vi "Remove RTDriver VIs.vi"(8 "error in (no error)":errorcluster, 11 ".NET Refnum in":refnum<k24>) -> (0 "error out":errorcluster, 3 ".NET Refnum out":refnum<k24>)   [LabVIEW 2019, in "TemplatePPL System Explorer.lvlib"]
uses:
  TemplatePPL System Explorer.lvlib
  NationalInstruments.VeriStand.SystemStorage
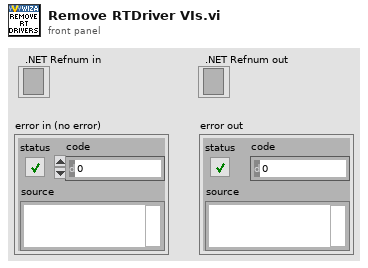
[diagram p1: front panel]
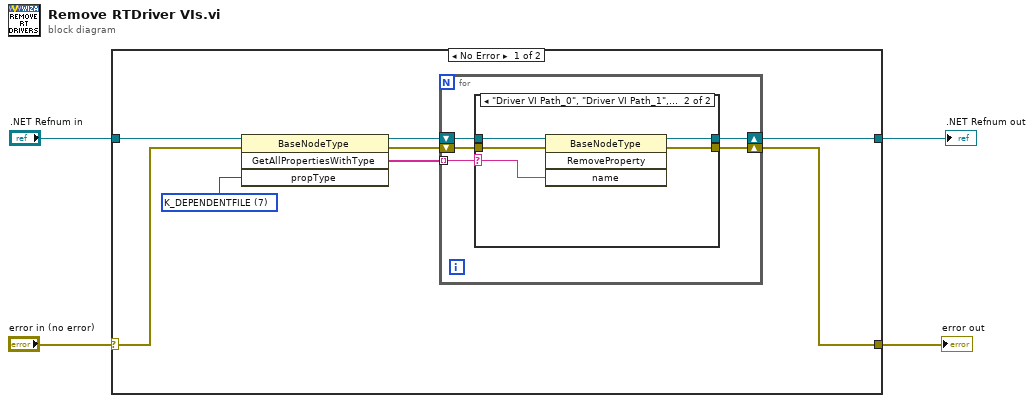
[diagram p0: block diagram]
diagram:
  n1 = case shown="No Error" "error in (no error)" {
    selector: "error in (no error)" -> [w7 w25]
    tunnel: [w12 w25] -> w4
    tunnel: [w11 w26] -> w1
    tunnel: ".NET Refnum in" -> [w8 w26]
    frame No Error {
      w9 = 7 items=["K_STRING", "K_BOOL", "K_I32", "K_U32", "K_DOUBLE", "K_U64", "K_VARIANT", "K_DEPENDENTFILE", "K_DEPENDENTNODE", "K_DATASOURCENODE", "K_U16", "K_DBLARR", "K_U32ARR", "K_I32ARR", "K_STRINGARR", "K_DICTIONARY", "K_DICTIONARYARR", "K_BINARYSTRING", "K_I16", "K_I64", "K_BOOLARR", "K_U64ARR", "K_U16ARR", "K_I64ARR", "K_I16ARR"] ("propType")
      n2 = invoke class="BaseNodeType" method="GetAllPropertiesWithType"(reference=w8, error in=w7, "propType"=w9) -> (reference out=w6:refnum<k24>, error out=w10:errorcluster, "GetAllPropertiesWithType"=w5:string[])  [unwired: 1 in, 1 out]
      n3 = for {
        tunnel: w5 -> [w13] mode=indexing
        shift-right: [w15] -> w12
        shift-left: w10 -> [w16]
        shift-right: [w14] -> w11
        shift-left: w6 -> [w17]
        n4 = case shown="\"Driver VI Path_0\", \"Driver VI Path_1\", \"Driver VI Path_2\", \"Driver VI Path_3\", \"Driver VI Path_4\"" w13 {
          selector: w13 -> [_ w20]
          tunnel: w17 -> [w19 w24]
          tunnel: w16 -> [w18 w23]
          tunnel: [w18 w22] -> w15
          tunnel: [w19 w21] -> w14
          frame "None", Default {
          }
          frame "Driver VI Path_0", "Driver VI Path_1", "Driver VI Path_2", "Driver VI Path_3", "Driver VI Path_4" {
            n5 = invoke class="BaseNodeType" method="RemoveProperty"(reference=w24, error in=w23, "name"=w20) -> (reference out=w21:refnum<k24>, error out=w22:errorcluster)  [unwired: 1 in, 2 out]
          }
        }
      }
    }
    frame Error {
    }
  }
  "error out" <- w4
  ".NET Refnum out" <- w1
